vi "Get Tamer Logo.vi"() -> (0 "Tamer Logo":picture)   [LabVIEW 2026, in "TALOS.lvlib"]
uses:
  TALOS.lvlib
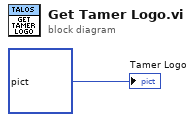
[diagram p0: block diagram]
diagram:
  "Tamer Logo" <- picture bytes[12830] ("Tamer Picture 2")
